vi "Get king square by color.vi"(10 "Color":T4, 11 "Board in":refnum<class "Board.lvclass">) -> (1 "Square":T1={"File"=enum."d", "Rank"=enum."4"}, 2 "found?":bool, 3 "Board out":refnum<class "Board.lvclass">)   [LabVIEW 2015, in "Chesslib.lvlib" / "Board.lvclass"]
uses:
  Board.lvclass
  typedef/Color.ctl
  typedef/Square.ctl
  typedef/File.ctl
  typedef/Rank.ctl
  Board.lvclass/Board.ctl
  typedef/Piece type.ctl
  Pieces/Piece/Piece.lvclass
  Chesslib.lvlib
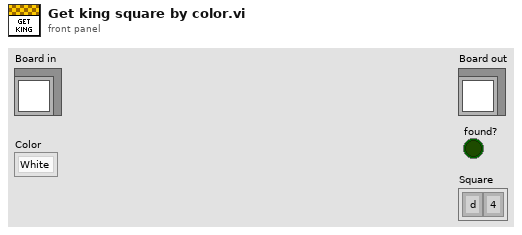
[diagram p1: front panel]
types:
  T1 = typedef "Chesslib.lvlib/Square.ctl" = cluster{"File":T2, "Rank":T3}
  T2 = typedef "Chesslib.lvlib/File.ctl" = enum16{"a", "b", "c", "d", "e", "f", "g", "h"}
  T3 = typedef "Chesslib.lvlib/Rank.ctl" = enum16{"1", "2", "3", "4", "5", "6", "7", "8"}
  T4 = typedef "Chesslib.lvlib/Color.ctl" = enum16{"White", "Black"}
  T5 = cluster{"Occupied":bool, "Piece":refnum<class "Piece.lvclass">}[]
  T6 = typedef "Chesslib.lvlib/Piece type.ctl" = enum16{"Pawn", "Bishop", "Knight", "Rook", "Queen", "King"}
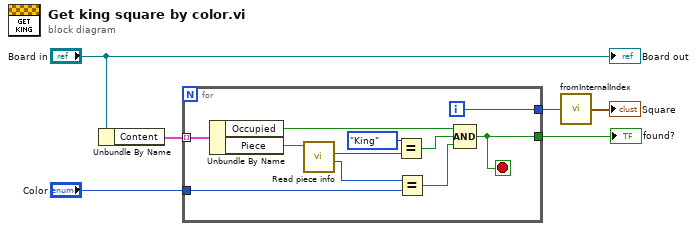
[diagram p0: block diagram]
diagram:
  n1 = Unbundle By Name("Board in") -> ("Content"=w6:T5)
  n2 = for {
    tunnel: w6 -> [w17] mode=indexing
    tunnel: "Color" -> [w13]
    tunnel: [w7] -> w2
    tunnel: [w8] -> w3
    i -> [w7]
    stop <- w8 stop-if-true
    n3 = Unbundle By Name(w17) -> ("Occupied"=w15:bool, "Piece"=w16:refnum<class "Piece.lvclass">)
    n4 = call "Read piece info.vi"("Piece in"=w16) -> ("Color"=w14:T4, "Piece type"=w11:T6)  [unwired: 9 in]
    n5 = Equal?(x=Piece_type."King", y=w11) -> (x = y?=w9:bool)
    n6 = Equal?(x=w14, y=w13) -> (x = y?=w12:bool)
    n7 = Compound Arithmetic op=AND(w15, w9, w12) -> (w8:bool)
  }
  "found?" <- w3
  n8 = call "fromInternalIndex.vi"("Internal index"=w2) -> ("Square"=→"Square":T1)
  "Board out" <- "Board in"
